vi "EvalRecFC-Data.vi"() -> ()   [LabVIEW 2012]
uses:
  <vilib>/Utility/file.llb/Read From Spreadsheet File (string).vi
panel:
  out "GPS Speed 2":cluster{dbl[], dbl[]}[](graph)
  out "selected path":path
  in  "Registerkarte":T1(tab)
  out "Tabellenelement":string[][](table)
  out "Gyro":cluster{dbl[], dbl[]}[](graph)
  out "GPS Speed":cluster{dbl[], dbl[]}(graph)
  out "ACC":cluster{dbl[], dbl[]}[](graph)
  out "Heading":cluster{dbl[], dbl[]}[](graph)
  out "Höhe":cluster{dbl[], dbl[]}[](graph)
  # "Legend"
  # "Altitude [m]"
  # "Min:     475\nMax:    525\nactual: 512"
  # "Heading [°]"
  # "Min:     0\nMax:    360\nactual: 193"
  # "Speed [km/h]"
  # "Min:     0\nMax:    123\nactual: 81"
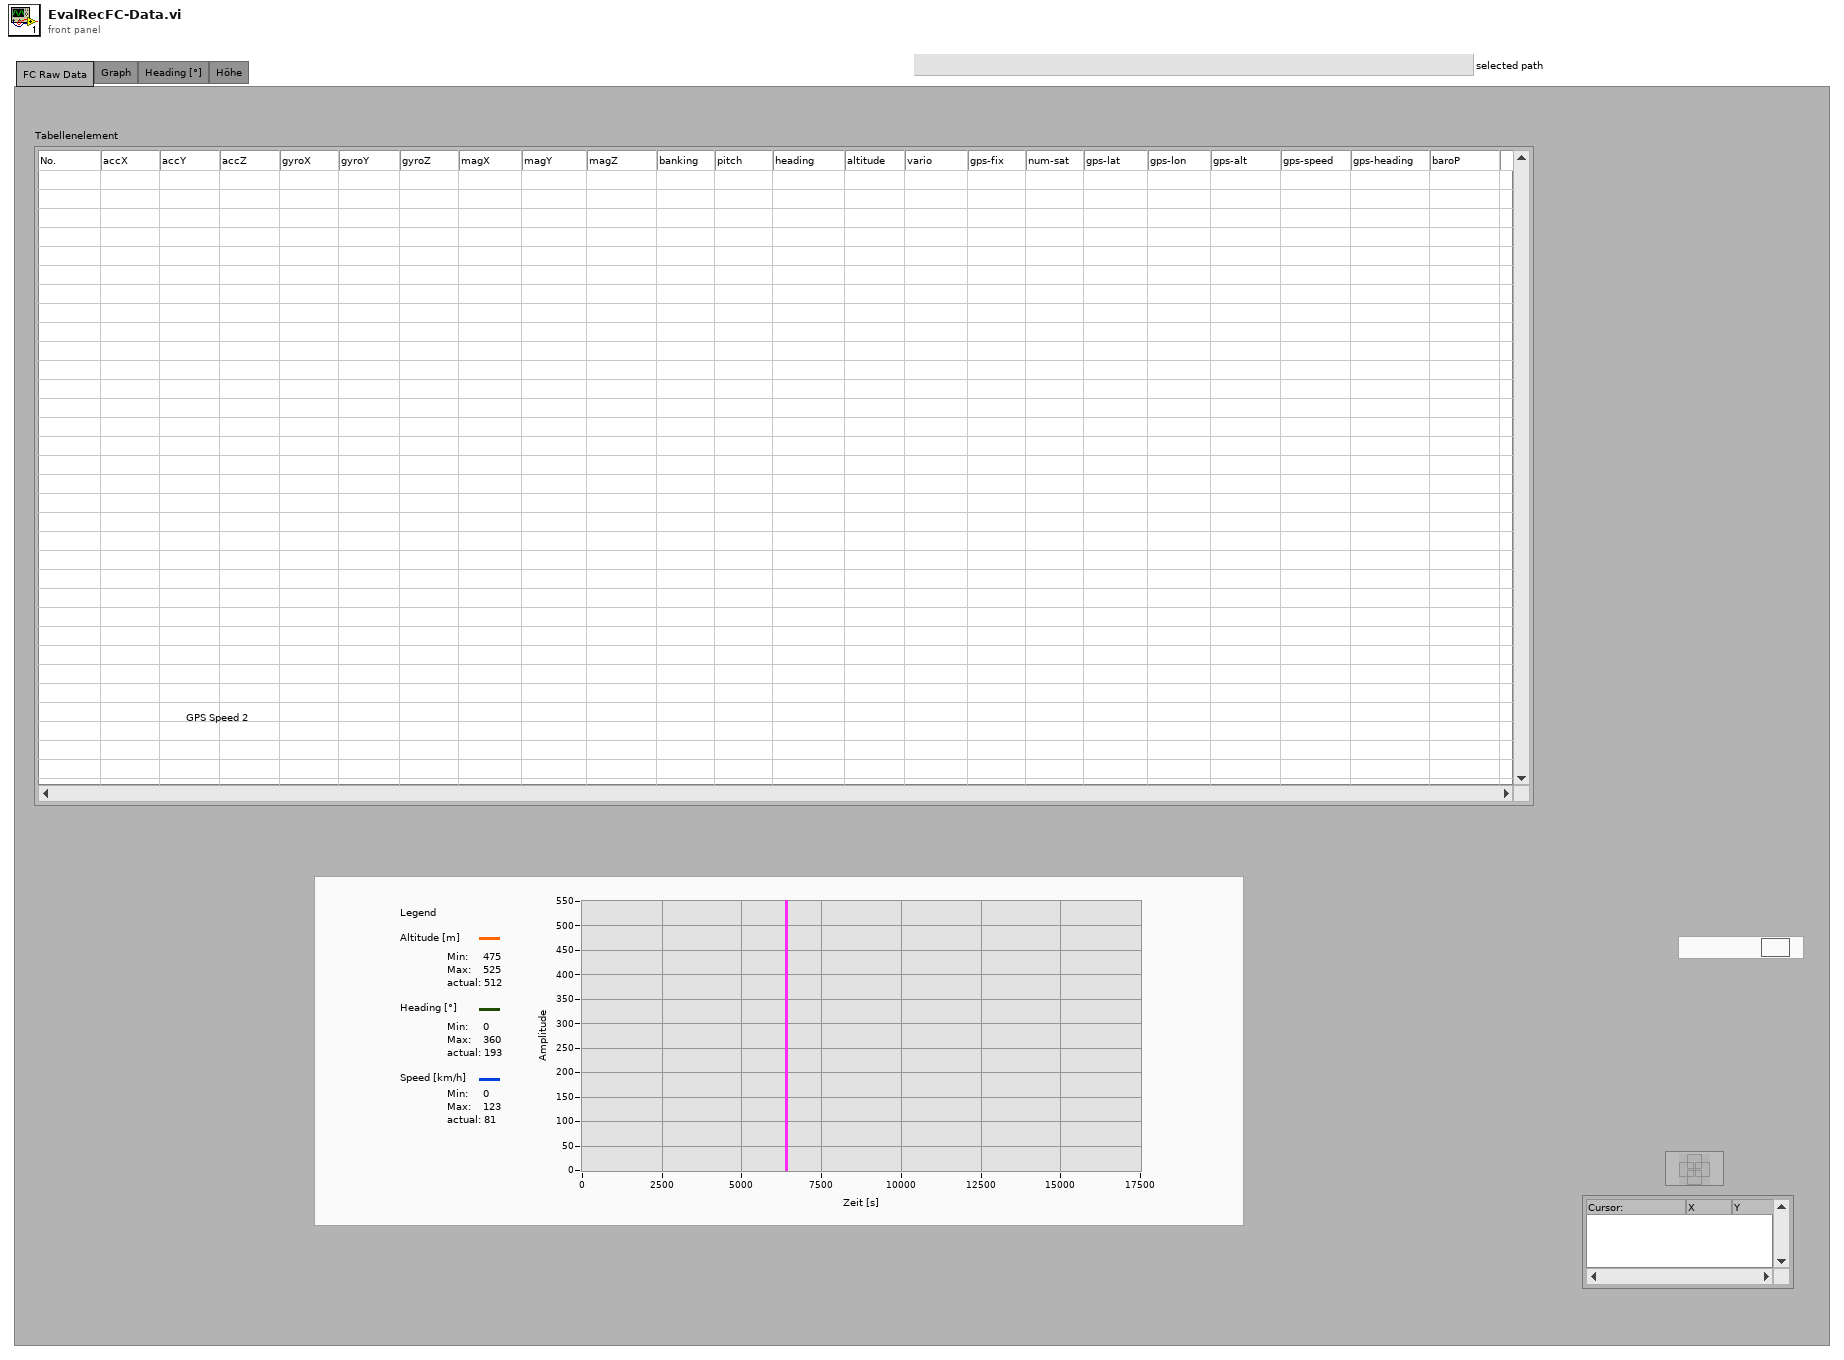
[diagram p1: front panel]
types:
  T1 = enum32{"FC Raw Data", "Graph", "Heading [°]", "Höhe"}
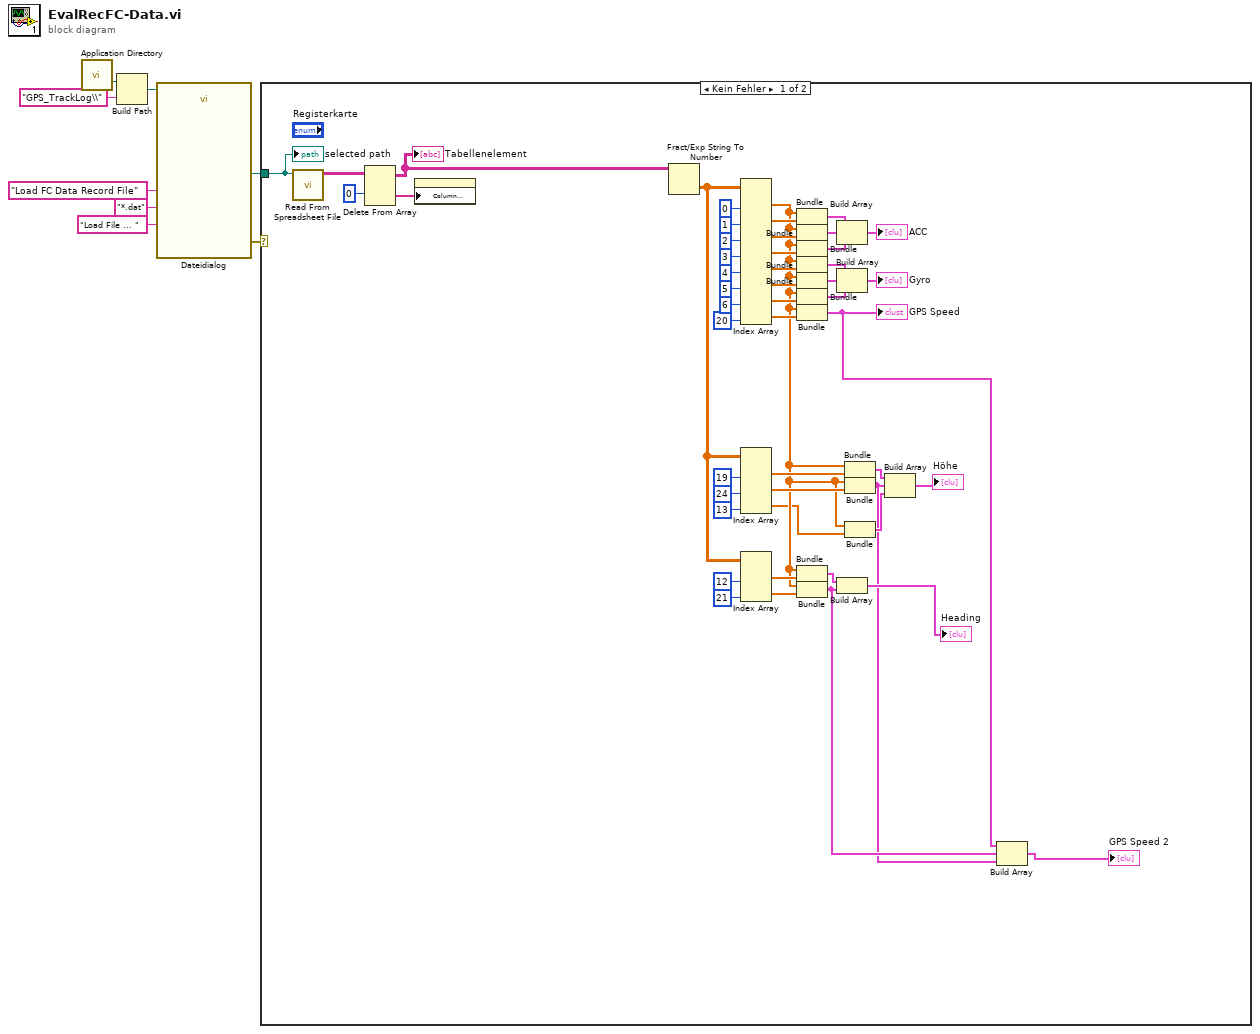
[diagram p0: block diagram]
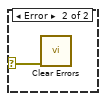
[diagram p2: hidden frame]
diagram:
  n1 = call <vilib>:"Application Directory.vi"() -> ("Application Directory"=w8:path)
  n2 = Build Path(base path=w8, name or relative path="GPS_TrackLog\\" ("String")) -> (appended path=w6:path)
  n3 = call "Dateidialog"("start path"=w6, "prompt"="Load FC Data Record File", "button label"="Load File ... ", "pattern (all files)"="*.dat") -> ("selected path"=w1:path, "error out"=w2:errorcluster)  [unwired: 8 in, 2 out]
  n4 = case shown="Kein Fehler" w2 {
    selector: w2 -> [_ w58]
    tunnel: w1 -> [w57 _]
    frame No Error {
      n5 = call-poly <vilib>:"Read From Spreadsheet File.vi"("file path (dialog if empty)"=w57) -> ("all rows"=w56:string[][])  [unwired: 6 in, 4 out]
      n6 = Delete From Array(array=w56, index (row)=0 ("Index (Zeile)")) -> (deleted portion=w54:string[], array with subset deleted=w53:string[][])  [unwired: 2 in]
      "Tabellenelement" <- w53
      n7 = property on="Tabellenelement" class="Tbl (strikt)"("Column Headers[]"=w54) -> ()  [unwired: 2 in, 2 out]
      n8 = Fract/Exp String To Number(string=w53) -> (number=w30:dbl[][])  [unwired: 3 in, 1 out]
      n9 = Index Array(array=w30, index (col) #1=0 ("Deaktivierter Index (Spalte)"), index (col) #2=1 ("Index (Spalte)"), index (col) #3=2 ("Index (Spalte)"), index (col) #4=3 ("Index (Spalte)"), index (col) #5=4 ("Index (Spalte)"), index (col) #6=5 ("Index (Spalte)"), index (col) #7=6 ("Index (Spalte)"), index (col) #8=20 ("Index (Spalte)")) -> (element #1=w15:dbl[], element #2=w42:dbl[], element #3=w48:dbl[], element #4=w43:dbl[], element #5=w22:dbl[], element #6=w21:dbl[], element #7=w20:dbl[], element #8=w17:dbl[])  [unwired: 8 in]
      n10 = Index Array(array=w30, index (col) #1=19 ("Deaktivierter Index (Spalte)"), index (col) #2=24 ("Index (Spalte)"), index (col) #3=13 ("Index (Spalte)")) -> (element #1=w39:dbl[], element #2=w38:dbl[], element #3=w13:dbl[])  [unwired: 3 in]
      n11 = Index Array(array=w30, index (col) #1=12 ("Deaktivierter Index (Spalte)"), index (col) #2=21 ("Index (Spalte)")) -> (element #1=w33:dbl[], element #2=w34:dbl[])  [unwired: 2 in]
      n12 = Bundle(w15, w42) -> (w52:cluster{dbl[], dbl[]})  [unwired: 1 in]
      n13 = Bundle(w15, w48) -> (w47:cluster{dbl[], dbl[]})  [unwired: 1 in]
      n14 = Bundle(w15, w43) -> (w45:cluster{dbl[], dbl[]})  [unwired: 1 in]
      n15 = Bundle(w15, w22) -> (w26:cluster{dbl[], dbl[]})  [unwired: 1 in]
      n16 = Bundle(w15, w21) -> (w27:cluster{dbl[], dbl[]})  [unwired: 1 in]
      n17 = Bundle(w15, w20) -> (w28:cluster{dbl[], dbl[]})  [unwired: 1 in]
      n18 = Bundle(w15, w17) -> (w12:cluster{dbl[], dbl[]})  [unwired: 1 in]
      "GPS Speed" <- w12
      n19 = Bundle(w15, w33) -> (w35:cluster{dbl[], dbl[]})  [unwired: 1 in]
      n20 = Bundle(w15, w34) -> (w11:cluster{dbl[], dbl[]})  [unwired: 1 in]
      n21 = Build Array(w52, w47, w45) -> (→"ACC":cluster{dbl[], dbl[]}[])
      n22 = Build Array(w26, w27, w28) -> (→"Gyro":cluster{dbl[], dbl[]}[])
      n23 = Build Array(w35, w11) -> (→"Heading":cluster{dbl[], dbl[]}[])
      n24 = Bundle(w15, w39) -> (w37:cluster{dbl[], dbl[]})  [unwired: 1 in]
      n25 = Bundle(w15, w38) -> (w9:cluster{dbl[], dbl[]})  [unwired: 1 in]
      n26 = Bundle(w15, w13) -> (w14:cluster{dbl[], dbl[]})  [unwired: 1 in]
      n27 = Build Array(w37, w9, w14) -> (→"Höhe":cluster{dbl[], dbl[]}[])
      n28 = Build Array(w12, w11, w9) -> (→"GPS Speed 2":cluster{dbl[], dbl[]}[])
      "selected path" <- w57
    }
    frame Error {
      n29 = call <vilib>:"Clear Errors.vi"("error in (no error)"=w58) -> ()  [unwired: 6 in, 1 out]
    }
  }
